vi "E2.vi"() -> ()   [LabVIEW 2014]
panel:
  out "IsWorking":bool
  in  "IsBleeding":bool
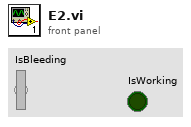
[diagram p1: front panel]
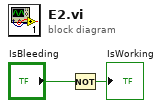
[diagram p0: block diagram]
diagram:
  n1 = Not(x="IsBleeding") -> (.not. x?=→"IsWorking":bool)
